vi "equalize_trajectory.vi"(8 "error in (no error)":errorcluster, 11 "ScanModeTS090821Circular2D in":refnum<class "ScanModeTS090821Circular2D.lvclass">=refnum) -> (0 "error out":errorcluster, 3 "ScanModeTS090821Circular2D out":refnum<class "ScanModeTS090821Circular2D.lvclass">)   [LabVIEW 2010]
uses:
  main/labview_source/type_definitions/classes/GenericTrajectory/GenericTrajectory.lvclass
  ScanModeTS090821Circular2D.lvclass
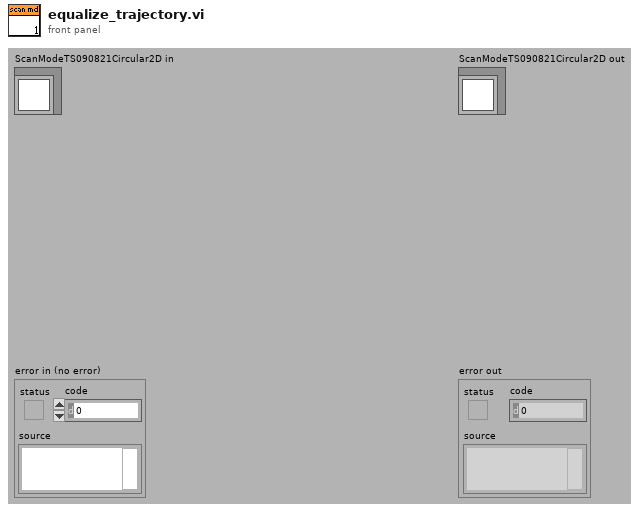
[diagram p1: front panel]
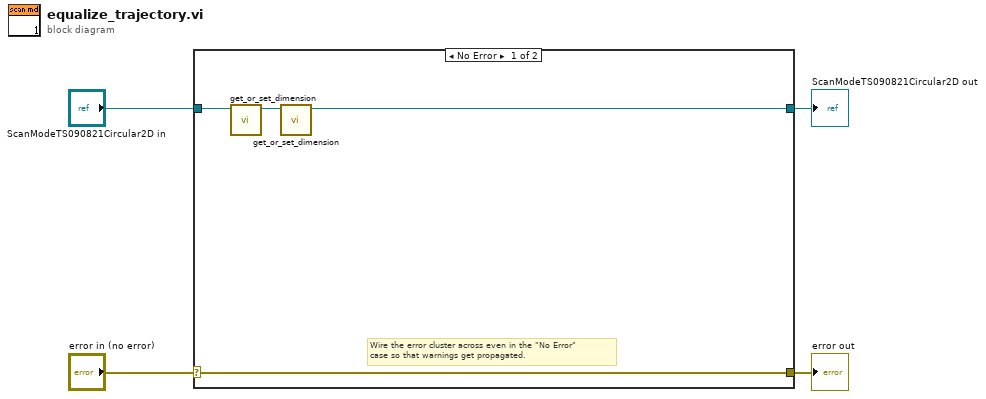
[diagram p0: block diagram]
diagram:
  n1 = case shown="No Error" "error in (no error)" {
    selector: "error in (no error)" -> [w8 w10]
    tunnel: [w8 w10] -> w3
    tunnel: [w6 w9] -> w1
    tunnel: "ScanModeTS090821Circular2D in" -> [w5 w9]
    frame No Error {
      # "Wire the error cluster across even in the \"No Error\"\ncase so that warnings get propagated."
      n2 = call-dynamic "get_or_set_dimension.vi"("GenericTrajectory in"=w5) -> ("GenericTrajectory out"=w7:refnum<class "GenericTrajectory.lvclass">)  [unwired: 8 in, 2 out]
      n3 = call-dynamic "get_or_set_dimension.vi"("GenericTrajectory in"=w7) -> ("GenericTrajectory out"=w6:refnum<class "GenericTrajectory.lvclass">)  [unwired: 8 in, 2 out]
    }
    frame Error {
    }
  }
  "error out" <- w3
  "ScanModeTS090821Circular2D out" <- w1
